vi "Read Transmission Data Unit.vi"(8 "error in":errorcluster, 11 "Modbus instance in":refnum<class "Modbus API.lvclass">) -> (0 "error out":errorcluster, 2 "transmission data unit":refnum<class "Transmission Data Unit.lvclass">, 3 "Modbus instance out":refnum<class "Modbus API.lvclass">)   [LabVIEW 2012, in "Modbus API.lvclass"]
doc: "This VI is an accessor for the transmission data unit stored in the Modbus instance. This accessor can be used as a property node. The transmission data unit is used by the device to determine how to pack and unpack data coming from the physical bus."
uses:
  Modbus API.lvclass
  Transmission Data Unit/Transmission Data Unit.lvclass
  Modbus API.lvclass/Modbus API.ctl
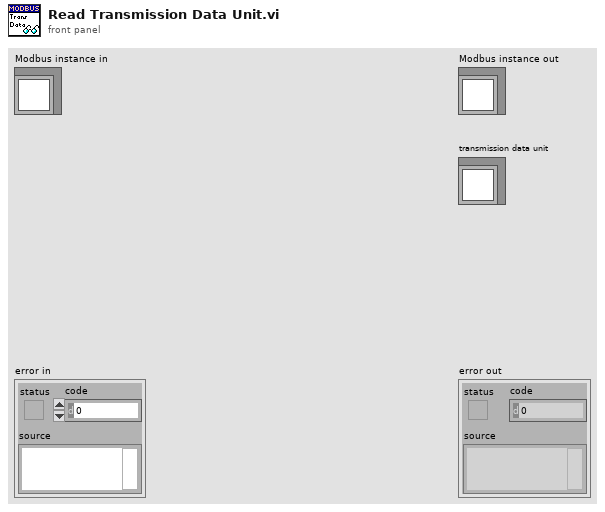
[diagram p1: front panel]
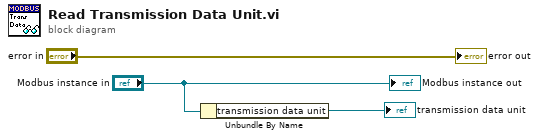
[diagram p0: block diagram]
diagram:
  n1 = Unbundle By Name("Modbus instance in") -> ("transmission data unit"=→"transmission data unit":refnum<class "Transmission Data Unit.lvclass">)
  "error out" <- "error in"
  "Modbus instance out" <- "Modbus instance in"
